vi "students-hardware.vi"() -> ()   [LabVIEW 2009]
doc: "This is a template VI for interfacing with the ECP Torsional Plant using an FPGA card."
uses:
  <vilib>/Analysis/Matrix/Datatypes/RealMatrix.ctl
  <vilib>/addons/Control Design/_Model Construction/Model Typedefs.llb/CD State Space Model (MIMO).ctl
  <vilib>/addons/Control Design/_Model Construction/Model Typedefs.llb/CD General Elements.ctl
  <vilib>/rvi/interface/nirviOpenFPGA/nirviOpenFPGA.xnode
  torsional-fpga-interface.lvbit
  <vilib>/FPGAPlugInAG/Pci-7831r/nirviIntfOpen_PCI-7831R.vi
  <vilib>/rvi/interface/nirviMethod/nirviMethod.xnode
  <vilib>/rvi/ClientSDK/nirviWhatTheDeviceIsDoing.ctl
  <vilib>/rvi/interface/common/niFpgaNodeNameForErrorReporting.ctl
  <vilib>/rvi/errors/niLvFpgaWhatHappensToTopLevelVI.ctl
  <vilib>/LabVIEW Targets/FPGA/Rio/nirio_HostInterface/nirio_CleanUpAfterDownload.vi
  <vilib>/LabVIEW Targets/FPGA/Rio/nirio_HostInterface/nirio_ConfigureBitstreamVersion.vi
  <vilib>/LabVIEW Targets/FPGA/Rio/nirio_HostInterface/nirio_ConfigureRegisterAddresses.vi
  <vilib>/LabVIEW Targets/FPGA/Rio/nirio_HostInterface/nirio_PrepareForDownload.vi
  <vilib>/rvi/errors/niLvFpgaErrorClusterFromErrorCode.vi
  <vilib>/rvi/errors/nirviReportUnexpectedCaseInternalError.vi
  <vilib>/rvi/errors/nirviReportUnexpectedCaseInternalError (String).vi
  <vilib>/rvi/errors/nirviReportUnexpectedCaseInternalError (U32).vi
  <vilib>/RVI Host/nirviSupport.llb/nirviErrorClusterFromErrorCode.vi
  <vilib>/LabVIEW Targets/FPGA/Rio/nirio_HostInterface/nirio_ReadBig.vi
  <vilib>/LabVIEW Targets/FPGA/Rio/nirio_HostInterface/nirio_IsItOKToDownload.vi
  <vilib>/LabVIEW Targets/FPGA/Rio/nirio_HostInterface/nirio_Download.vi
  <vilib>/LabVIEW Targets/FPGA/Rio/nirio_HostInterface/nirio_DMAStopAll.vi
  <vilib>/LabVIEW Targets/FPGA/Rio/nirio_HostInterface/nirio_DisableInterrupts.vi
  <vilib>/Utility/error.llb/Error Cluster From Error Code.vi
  <vilib>/LabVIEW Targets/FPGA/Rio/nirio_HostInterface/nirio_Reset.vi
  <vilib>/rvi/errors/niLvFpgaReportInternalErrorWithAdditionalInfo.vi
  <vilib>/LabVIEW Targets/FPGA/Rio/nirio_HostInterface/nirio_DMAReconfigureDriver.vi
  <vilib>/LabVIEW Targets/FPGA/Rio/nirio_HostInterface/nirio_EnableInterrupts.vi
  <vilib>/LabVIEW Targets/FPGA/Rio/nirio_HostInterface/nirio_GetCompilationResults.vi
  <vilib>/rvi/FIFO/Fifo_Types/Fifo_DMA_Config.ctl
  <vilib>/rvi/DataTransferAndStorage/Container/Common/niFpgaDataTypeControl.ctl
  <vilib>/rvi/ClientSDK/Core/ModuleGeneration/CommunicationInterfaceUtility/niFpgaDmaChannelImplementation.ctl
  <vilib>/rvi/errors/niLvFpgaAdjustHostInterfaceError.vi
  <vilib>/rvi/interface/nirviReadWriteControl/nirviReadWriteControl.xnode
  <vilib>/Simulation/Scripting/Companion Diagram/SimConfigNode/SimDog.xnode
  <vilib>/Simulation/Scripting/Companion Diagram/SimConfigNode/SimParams.ctl
  <vilib>/Simulation/Scripting/Companion Diagram/SimConfigNode/_simSolvers.ctl
  <vilib>/Simulation/Implementation/Shared/SIMSCR Execution Mode.ctl
  <vilib>/Utility/file.llb/Write To Spreadsheet File (DBL).vi
  <vilib>/Simulation/Implementation/Shared/SIM Bundle Sim Info.vi
  <vilib>/Simulation/Implementation/Shared/NILVSim_GetModelError.vi
  <vilib>/Simulation/Implementation/Shared/SIM Unbundle Sim Info.vi
  <vilib>/Platform/TimedLoop/XDataNode/XDataNode.xnode
  <vilib>/Platform/TimedLoop/XDataNode/loadlvalarms.vi
  <vilib>/Platform/TimedLoop/XDataNode/timing_clust.ctl
  <vilib>/Platform/TimedLoop/XDataNode/nitl_modes.ctl
  <vilib>/Platform/TimedLoop/XDataNode/wakeup.ctl
  <vilib>/Simulation/Implementation/Shared/NILVSim_Initialize.vi
  <vilib>/Simulation/Implementation/Shared/NILVSim_FinishedLate.vi
  <vilib>/Simulation/Implementation/Shared/NILVSim_Manager.vi
  <vilib>/Simulation/Scripting/Editor Utilities/SIM subVI tag data.ctl
  <vilib>/Simulation/Scripting/Editor Utilities/SIM subVI execution type.ctl
  <vilib>/Simulation/DataSources/SIMX PulseGenerator/SIMX PulseGenerator.xnode
  <vilib>/Simulation/DataSources/Implementation/NILVSim Pulse Generator.llb/SIM Pulse Generator (scalar).vi
  <vilib>/Simulation/Utility/SIMX Halt/SIMX Halt.xnode
  <vilib>/Simulation/Utility/Implementation/SIM Halt.vi
  <vilib>/Simulation/ContinuousLinear/Implementation/NILVSim State Space.llb/SIM State Space Collector (CD).vi
  <vilib>/Simulation/Implementation/Shared/SIM Fire Discrete SubVI.vi
  <vilib>/Simulation/ContinuousLinear/Implementation/NILVSim State Space.llb/SIM State Space Distributor (CD).vi
  <vilib>/Simulation/SignalArithmetic/SIMX Gain/SIMX Gain.xnode
  <vilib>/Simulation/SignalArithmetic/Implementation/NILVSim Gain.llb/SIM Gain (vector,MatrixGain).vi
  <vilib>/Simulation/SignalArithmetic/Implementation/NILVSim Gain.llb/SIM Gain (scalar).vi
  <vilib>/Simulation/SignalArithmetic/SIMX Summation/SIMX Summation.xnode
  <vilib>/Simulation/Utility/SIMX Collector/SIMX Collector.xnode
  <vilib>/Simulation/Utility/Implementation/NILVSim Collector.llb/SIM Collector (scalar).vi
  <vilib>/Simulation/SignalDisplay/SIMX TimeWaveform/SIMX TimeWaveform.xnode
  <vilib>/Simulation/SignalDisplay/Implementation/NILVSim Time Waveform.llb/SIM Time Waveform (scalar).vi
  <vilib>/Simulation/SignalDisplay/Implementation/NILVSim Time Waveform.llb/SIM Time Waveform (vector).vi
  <vilib>/Simulation/Implementation/Shared/NILVSim_FinalizeModel.vi
  <vilib>/rvi/interface/nirviCloseFPGA/nirviCloseFPGA.xnode
  <vilib>/FPGAPlugInAG/Pci-7831r/nirviIntfClose_PCI-7831R.vi
  <vilib>/Simulation/ContinuousLinear/SIMX StateSpace/SIMX StateSpace.xnode
  <vilib>/userDefined/High Color/nirio_resource_hc.ctl
  NiRioSrv.dll
  <vilib>/Simulation/ContinuousLinear/Implementation/NILVSim State Space.llb/SIM State Space (CD).vi
  <vilib>/Platform/TimedLoop/XDataNode/XDNodeRunTimeDep.lvlib
  <vilib>/Analysis/Matrix/NI_Matrix.lvlib
  <vilib>/addons/Control Design/_Model Construction/NI_LinSys_Model Typedefs.lvlib
panel:
  out "Killswitch Activated":bool
  in  "Loop Period (ms)":i32=5 min=1 max=100
  out "Estimator":T1 {"Transport Delay" format="%.2f"; "D" format="%#.2g"; "C" format="%#.2g"; "B" format="%#.2g"; "A" format="%#.2g"; "properties"."Sampling Time" format="%#.6p"; "properties"."Output Delays" format="%.4f"; "properties"."Input Delays" format="%.4f"}
  out "K":T3
  out "Nbar":dbl
  out "Torque Output":waveform(dbl)(graph)
  out "Angles":waveform(dbl)[](graph)
  out "Sample Rate (Hz)":dbl
  in  "Abort":bool
  in  "Final Time (s)":dbl=30.0 min=1.0 step=0.01
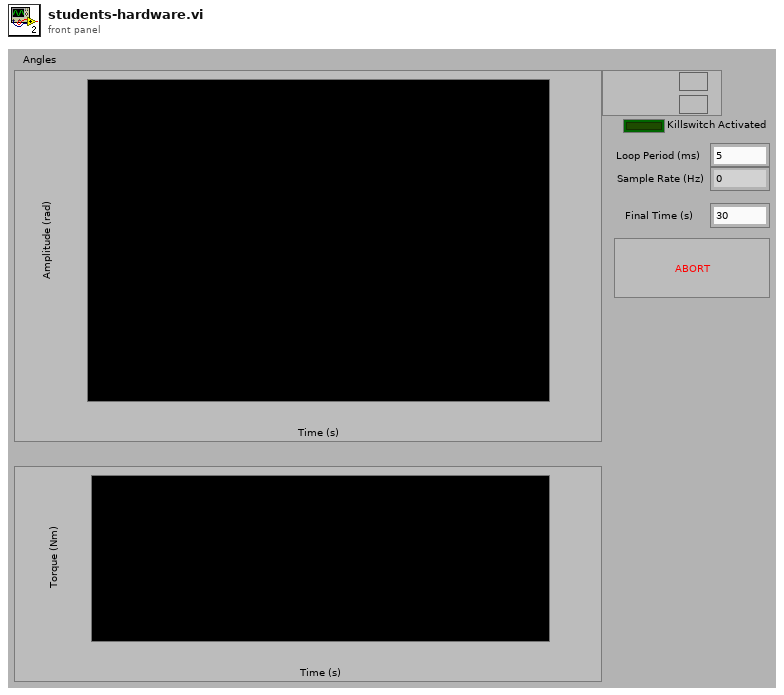
[diagram p1: front panel]
types:
  T1 = typedef "NI_LinSys_Model Typedefs.lvlib/CD State Space Model (MIMO).ctl" = cluster{"properties":T2, "A":dbl[][], "B":dbl[][], "C":dbl[][], "D":dbl[][], "StateNames":string[], "Transport Delay":dbl[][]}
  T2 = typedef "NI_LinSys_Model Typedefs.lvlib/CD General Elements.ctl" = cluster{"Model name":string, "Input names":string[], "Output names":string[], "Input Delays":dbl[], "Output Delays":dbl[], "Sampling Time":dbl, "Notes":string}
  T3 = typedef "NI_Matrix.lvlib/RealMatrix.ctl" = dbl[][]
  T4 = typedef "niFpgaNodeNameForErrorReporting.ctl" = enum16{"Open FPGA VI Reference", "Read/Write Control", "Invoke Method: Abort", "Invoke Method: Acknowledge IRQ", "Invoke Method: Download", "Invoke Method: FIFO.Configure", "Invoke Method: FIFO.Read", "Invoke Method: FIFO.Start", "Invoke Method: FIFO.Stop", "Invoke Method: FIFO.Write", "Invoke Method: Reset", "Invoke Method: Run", "Invoke Method: Wait on IRQ", "Close FPGA VI Reference"}
  T5 = typedef "niLvFpgaWhatHappensToTopLevelVI.ctl" = enum16{"top level VI scripted behind XNode", "top level VI inlined behind XNode"}
  T6 = typedef "SIM subVI tag data.ctl" = cluster{"period":dbl, "skew":dbl, "Simulation execution type":T7}
  T7 = typedef "SIM subVI execution type.ctl" = enum16{"Function call", "Discrete", "Continuous", "Initialization only", "Final step only"}
  T8 = typedef "XDNodeRunTimeDep.lvlib/timing_clust.ctl" = cluster{"Expected End [f-1]":u64, "Actual End [f-1]":u64, "Finished Late? [f-1]":bool, "Expected End [i-1]":u64, "Actual End [i-1]":u64, "Finished Late? [i-1]":bool, "Expected Start [i]":u64, "Actual Start [i]":u64, "Expected Start [f]":u64, "Actual Start [f]":u64, "Source Name":string, "Structure Name":string, "Period":i64, "Deadline":i64, "Offset":i64, "Start":i64, "Priority":i32, "Timeout":i32, "Mode":T9, "Wakeup Reason":T10, "Error":errorcluster, "Source Type":string, "Secondary Source Type":string, "Global End Time":u64, "Global Start Time":u64, "Frame Duration":u64, "Iteration Duration":u64, "Assigned CPU":i32, "I/O Scan Engine Mode":u32}
  T9 = typedef "XDNodeRunTimeDep.lvlib/nitl_modes.ctl" = enum32{"No Change", "Process missed periods, maintain original phase", "Discard missed periods, maintain original phase", "Process missed periods, ignore original phase", "Discard missed periods, ignore original phase"}
  T10 = typedef "XDNodeRunTimeDep.lvlib/wakeup.ctl" = enum32{"Normal", "Aborted", "Asynchronous wakeup", "Timing source error", "Timed loop error", "Timeout"}
  T11 = typedef "SimParams.ctl" = cluster{"Initial Time (s)":dbl, "Final Time (s)":dbl, "Step Size (s)":dbl, "ODE Solver":T12, "Minimum Step Size (s)":dbl, "Maximum Step Size (s)":dbl, "Relative Tolerance":dbl, "Absolute Tolerance":dbl, "Software Timing":bool, "Initial Step Size (s)":dbl, "Automatic Fixed Step Size?":bool, "Automatic Discrete Step Size?":bool, "Discrete Step Size (s)":dbl, "Calculate using Time Step":bool, "Solver Wired?":bool, "Prev.Frm.Expected End":u64, "Prev.Frm.Actual End":u64, "Prev.Frm.Finished Late?":bool, "Prev.Iter.Expected End":u64, "Prev.Iter.Actual End":u64, "Prev.Iter.Finished Late?":bool, "Expected Iteration Start":u64, "Actual Iteration Start":u64, "Expected Frame Start":u64, "Actual Frame Start":u64, "Source Name":string, "Name":string, "Period":i64, "Deadline":i64, "Offset":i64, "Start":i64, "Priority":i32, "Timeout":i32, "Processor":i32, "Mode":enum32{"No Change", "Process missed periods, maintain original phase", "Discard missed periods, maintain original phase", "Process missed periods, ignore original phase", "Discard missed periods, ignore original phase"}, "Wakeup reason":enum32{"Normal", "Aborted", "Asynchronous wakeup", "Timing source error", "Timed loop error", "Timeout"}, "Error":errorcluster, "Source Type":string, "Secondary Source Type":string, "Global End Time":u64, "Global Start Time":u64, "Full Solver Reset":bool, "Execution Mode":T13, "Nan/Inf Check":bool, "Custom Solver Library":string, "Solver Is Variable":bool, "custom solver name":string}
  T12 = typedef "_simSolvers.ctl" = enum16{"Runge-Kutta 1 (Euler)", "Runge-Kutta 2", "Runge-Kutta 3", "Runge-Kutta 4", "Runge-Kutta 23 (variable)", "Runge-Kutta 45 (variable)", "BDF (variable)", "Adams-Moulton (variable)", "Rosenbrock (variable)", "Discrete States Only", "Linearizer", "State Query", "Trim Eval", "Custom Solver"}
  T13 = typedef "SIMSCR Execution Mode.ctl" = u16
  T14 = cluster{"signature":u8[], "vi signatures match":bool, "signature register address":u32, "reset register address":u32, "control register address":u32, "interrupt base address":u32, "Bitstream Version":u32, "DMA Configuration":cluster{"Name":string, "Depth":u32, "Write? (Deprecated:Use Implementation)":bool, "Physical Channel":u32, "Base Address":u32, "Data Width":u32, "Data Type":enum32{"Boolean", "I8", "I16", "I32", "I64", "U8", "U16", "U32", "U64", "FXP"}, "FXP Properties":variant, "Write Window Address":u32, "Implementation":enum16{"niFpgaTargetToHost", "niFpgaHostToTarget", "niFpgaPeerToPeerWriter", "niFpgaPeerToPeerReader", "niCoreTargetToHost", "niCoreHostToTarget"}, "Control Set":u32}[], "run when loaded?":bool, "reset register size in bits":u32, "compilation results xml":string}
  T15 = typedef "nirviWhatTheDeviceIsDoing.ctl" = enum32{"nothing", "something other than LabVIEW FPGA", "FPGA interface", "interactive", "emulation"}
  T16 = typedef "Fifo_DMA_Config.ctl" = cluster{"Name":string, "Depth":u32, "Write? (Deprecated:Use Implementation)":bool, "Physical Channel":u32, "Base Address":u32, "Data Width":u32, "Data Type":T17, "FXP Properties":variant, "Write Window Address":u32, "Implementation":T18, "Control Set":u32}
  T17 = typedef "niFpgaDataTypeControl.ctl" = enum32{"Boolean", "I8", "I16", "I32", "I64", "U8", "U16", "U32", "U64", "FXP"}
  T18 = typedef "niFpgaDmaChannelImplementation.ctl" = enum16{"niFpgaTargetToHost", "niFpgaHostToTarget", "niFpgaPeerToPeerWriter", "niFpgaPeerToPeerReader", "niCoreTargetToHost", "niCoreHostToTarget"}
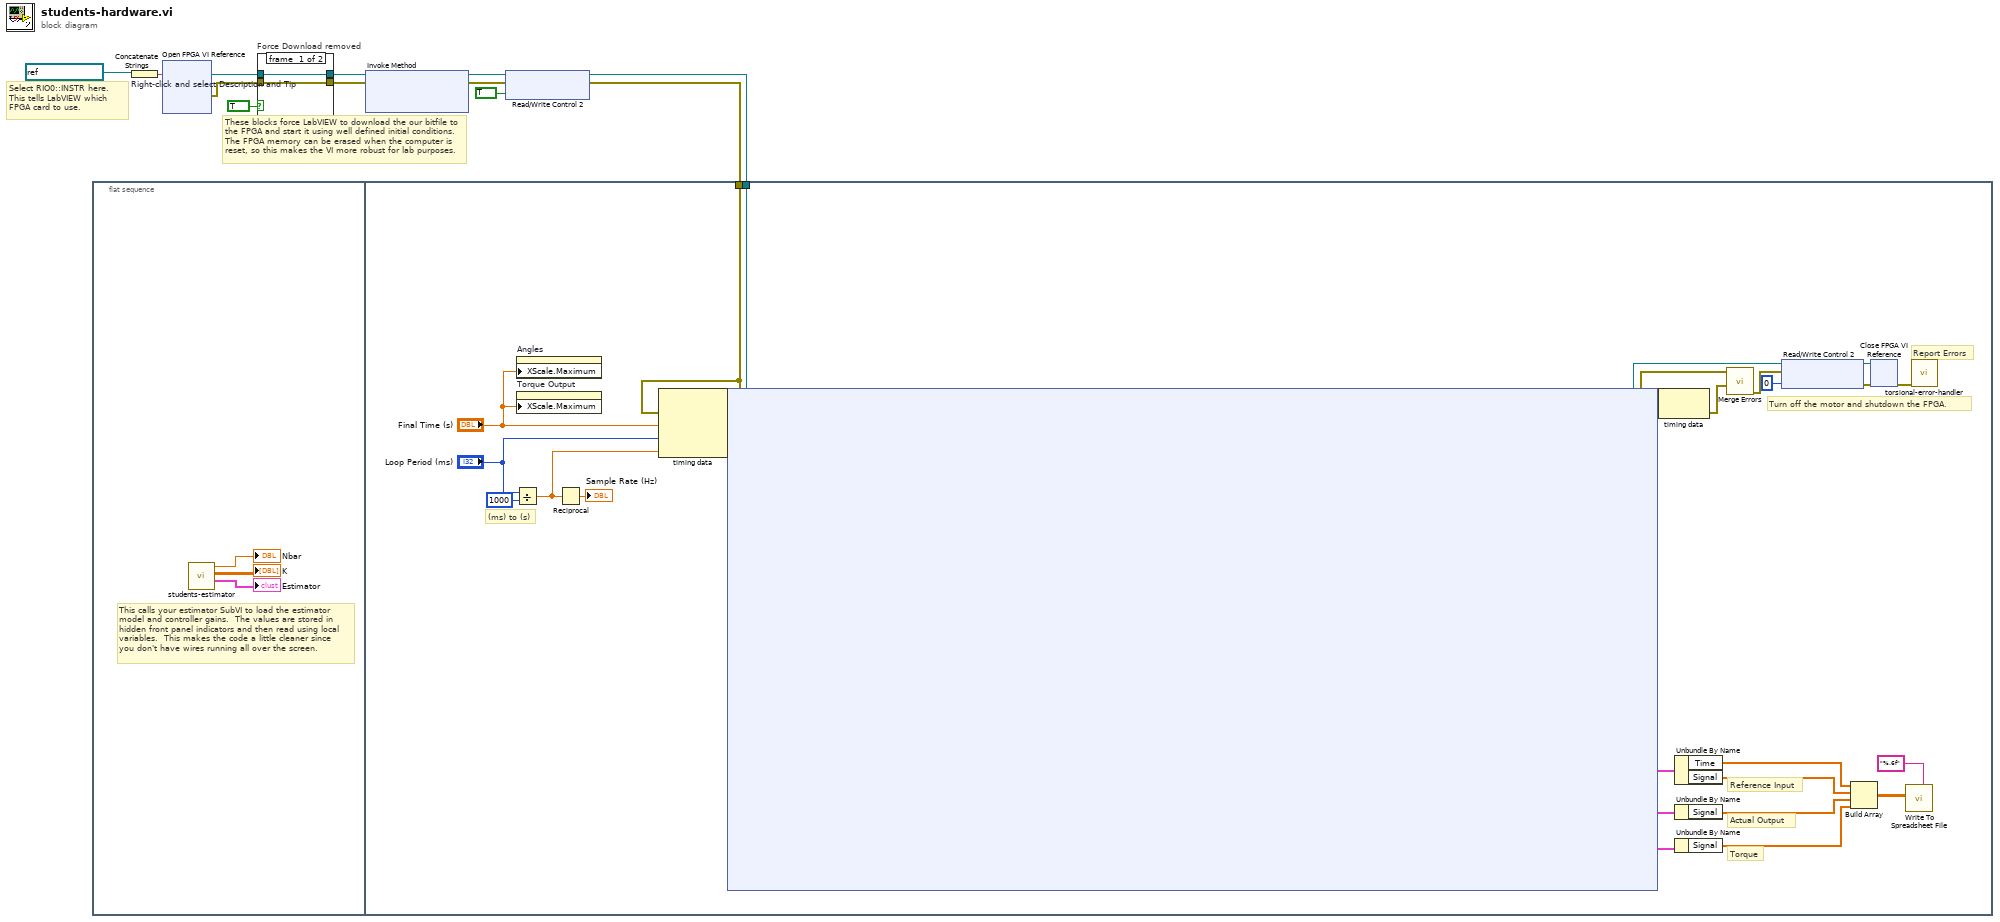
[diagram p0: block diagram]
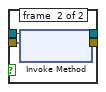
[diagram p2: hidden frame]
diagram:
  # "These blocks force LabVIEW to download the our bitfile to the FPGA and start it using well defined initial conditions.  The FPGA memory can be erased when the computer is reset, so this makes the VI more robust for lab purposes."
  # "Select RIO0::INSTR here.  This tells LabVIEW which FPGA card to use."
  n1 = flat-sequence {
    tunnel: w3 -> [w34]
    tunnel: w2 -> [w16]
    frame #0 {
      # "This calls your estimator SubVI to load the estimator model and controller gains.  The values are stored in hidden front panel indicators and then read using local variables.  This makes the code a little cleaner since you don't have wires running all over the screen."
      n2 = call "students-estimator.vi"() -> ("Estimator State Space Object"=→"Estimator":T1, "State Feedback Gain (K)"=→"K":T3, "Input Scaling (Nbar)"=→"Nbar":dbl)  [unwired: 1 out]
    }
    frame #1 {
      # "Actual Output"
      # "Reference Input"
      # "Torque"
      # "(ms) to (s)"
      # "Report Errors"
      # "Turn off the motor and shutdown the FPGA."
      n3 = Divide(x="Loop Period (ms)", y=1000) -> (x/y=w27:dbl)
      n4 = property on="Angles" class="WFChart (strict)"("XScale.Maximum"="Final Time (s)") -> ()  [unwired: 2 in, 2 out]
      n5 = property on="Torque Output" class="WFChart (strict)"("XScale.Maximum"="Final Time (s)") -> ()  [unwired: 2 in, 2 out]
      n6 = Reciprocal(x=w27) -> (1/x=→"Sample Rate (Hz)":dbl)
      n7 = node-c288(w16, "Final Time (s)", "Loop Period (ms)", w27) -> (w41:variant)
      n8 = node-c254 ("Control & Simulation Loop")(w41, w16, w34) -> (w40:variant, w32:refnum<k20>, w31:errorcluster, w26:cluster{"Time":dbl[], "Signal":dbl[]}, w25:cluster{"Time":dbl[], "Signal":dbl[]}, w24:cluster{"Time":dbl[], "Signal":dbl[]})
      n9 = node-c288(w40) -> (w30:errorcluster)
      n10 = Unbundle By Name(w26) -> ("Time"=w23:dbl[], "Signal"=w22:dbl[])
      n11 = Unbundle By Name(w25) -> ("Signal"=w20:dbl[])
      n12 = Unbundle By Name(w24) -> ("Signal"=w21:dbl[])
      n13 = call <vilib>:"Merge Errors.vi"("error in 3 (no error)"=w30, "error in 1 (no error)"=w31) -> ("error out"=w33:errorcluster)  [unwired: 5 in]
      n14 = xnode ("Read/Write Control 2")("FPGA VI Reference In"=w32, "error in"=w33, "Motor Voltage"=i16 0 ("Analog Out")) -> ("FPGA VI Reference Out"=w39:refnum<k20>, "error out"=w37:errorcluster)
      n15 = Build Array(w23, w22, w20, w21) -> (w19:dbl[][])
      n16 = xnode ("Close FPGA VI Reference")("FPGA VI Reference In"=w39, "error in"=w37) -> ("error out"=w36:errorcluster)
      n17 = call-poly <vilib>:"Write To Spreadsheet File.vi"("format (%.3f)"="%.6f", "2D data"=w19) -> ()  [unwired: 6 in, 1 out]
      n18 = call "torsional-error-handler.vi"("error in"=w36) -> ()  [unwired: 4 in]
    }
  }
  n19 = Concatenate Strings "Right-click and select Description and Tip"(refnum<visa-resource-name> "RIO0::INSTR" ("resource name")) -> (w1:string)
  n20 = xnode "Open FPGA VI Reference"("resource name"=w1) -> ("FPGA VI Reference Out"=w7:refnum<k20>, "error out"=w9:errorcluster)  [unwired: 1 in]
  n21 = case "Force Download removed" shown="True" TRUE ("Force Download (F)") {
    tunnel: w7 -> [w764 w768]
    tunnel: [w764 w767] -> w6
    tunnel: w9 -> [w763 w766]
    tunnel: [w763 w765] -> w4
    frame #0 {
    }
    frame #1 {
      n22 = xnode "Invoke Method"("FPGA VI Reference In"=w768, "error in"=w766) -> ("FPGA VI Reference Out"=w767:refnum<k20>, "error out"=w765:errorcluster)
    }
  }
  n23 = xnode "Invoke Method"("FPGA VI Reference In"=w6, "error in"=w4) -> ("FPGA VI Reference Out"=w12:refnum<k20>, "error out"=w8:errorcluster)  [unwired: 1 in]
  n24 = xnode ("Read/Write Control 2")("FPGA VI Reference In"=w12, "error in"=w8, "Reset Encoders"=TRUE) -> ("FPGA VI Reference Out"=w3:refnum<k20>, "error out"=w2:errorcluster)
